vi "mxwScript_Cmnd2Str_openTemplate.vi"(8 "error in (no error)":errorcluster, 11 "data":variant) -> (0 "error out":errorcluster, 3 "outputString":string)   [LabVIEW 2017]
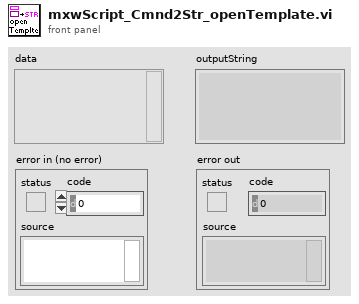
[diagram p1: front panel]
types:
  T1 = cluster{"location":string, "options":cluster{"option":string, "value":variant}[]}
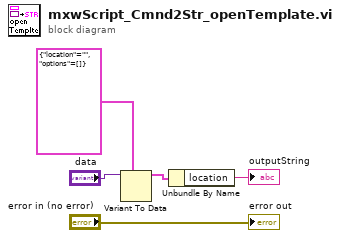
[diagram p0: block diagram]
diagram:
  n1 = Variant To Data(type=T1 {"location"="", "options"=[]}, Variant="data") -> (data=w2:T1)  [unwired: 1 in, 1 out]
  n2 = Unbundle By Name(w2) -> ("location"=→"outputString":string)
  "error out" <- "error in (no error)"
